vi "Update Display.vi"(8 "error in (no error)":errorcluster, 11 "English Picker in":refnum<class "English Picker.lvclass">) -> (0 "error out":errorcluster, 3 "English Picker out":refnum<class "English Picker.lvclass">)   [LabVIEW 2020, in "English Picker.lvlib" / "English Picker.lvclass"]
uses:
  English Picker.lvclass
  D:/Storage/Source Code/Clase AF/ClaseAF/05 AF Camera/Products Picker/Products Picker.lvclass
  Products Picker/Products Picker.lvclass/Products Picker.ctl
  English Picker.lvclass/English Picker.ctl
  Products Picker/Products Picker.lvclass
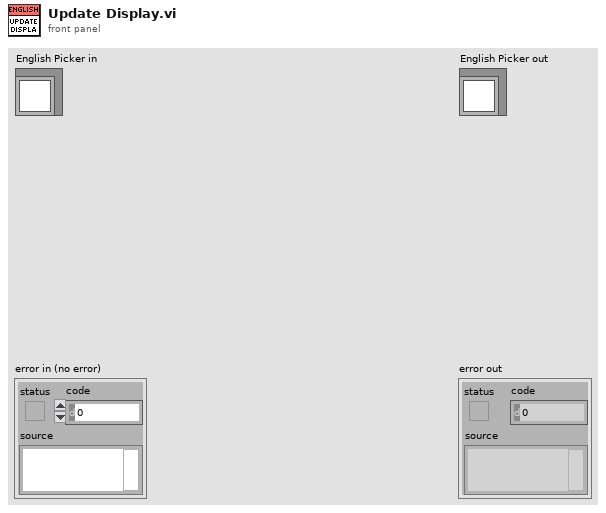
[diagram p1: front panel]
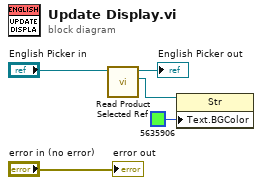
[diagram p0: block diagram]
diagram:
  n1 = call "Read Product Selected Ref.vi"("Products Picker in"="English Picker in") -> ("Product Selected Ref"=w2:refnum<vi>, "Products Picker out"=→"English Picker out":refnum<class "English Picker.lvclass">)  [unwired: 9 in]
  n2 = property on="Property Node" class="Str"(reference=w2, "Text.BGColor"=u32 5635906) -> ()  [unwired: 1 in, 2 out]
  "error out" <- "error in (no error)"
